vi "Error Message.vi"() -> (2 "Error":string)   [LabVIEW 2015]
uses:
  Galobal variable_TI.vi
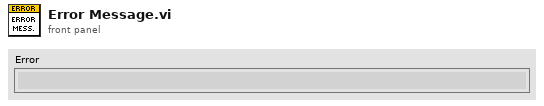
[diagram p1: front panel]
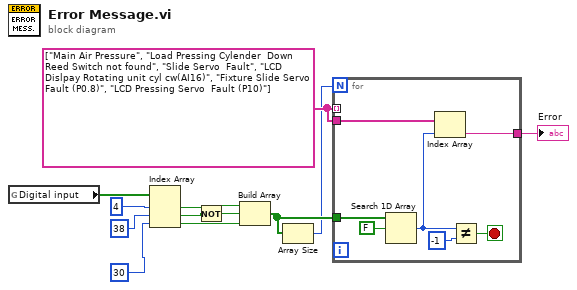
[diagram p0: block diagram]
diagram:
  w7 = string[] ["Main Air Pressure", "Load Pressing Cylender  Down Reed Switch not found", "Slide Servo  Fault", "LCD Dislpay Rotating unit cyl cw(AI16)", "Fixture Slide Servo Fault (P0.8)", "LCD Pressing Servo  Fault (P10)"]
  n1 = global read "Galobal variable_TI.vi" "Digital input"() -> (w12:bool[])
  n2 = Index Array(array=w12, index #1=4 ("index"), index #2=38 ("index"), index #3=30 ("index")) -> (element #1=w9:bool, element #2=w8:bool, element #3=w1:bool)
  n3 = Not(x=w8) -> (.not. x?=w3:bool)
  n4 = Build Array(w9, w3, w1) -> (w5:bool[])
  n5 = Array Size(array=w5) -> (size(s)=w4:i32)
  n6 = for {
    N: w4 -> [_]
    tunnel: w7 -> [_] mode=indexing
    tunnel: w7 -> [w15]
    tunnel: w5 -> [w17]
    tunnel: [w13] -> w6
    stop <- w16 stop-if-true
    n7 = Search 1D Array(1D array=w17, element=FALSE) -> (index of element=w14:i32)  [unwired: 1 in]
    n8 = Index Array(array=w15, index=w14) -> (element=w13:string)
    n9 = Not Equal?(x=w14, y=-1) -> (x != y?=w16:bool)
  }
  "Error" <- w6
